vi "ROOT - Restore Session Defaults.vi"(0 "Session Handle in":T1, 11 "error in (no error)":errorcluster) -> (4 "Session Handle out":T1, 15 "error out":errorcluster)   [LabVIEW 2017, in "Session - Root.lvclass"]
doc: "Initializes a measurement session\n\nSession data is set to the default values from \"set Defaults.vi\""
uses:
  Session - Root.lvclass
  Typedefs/Session Handle.ctl
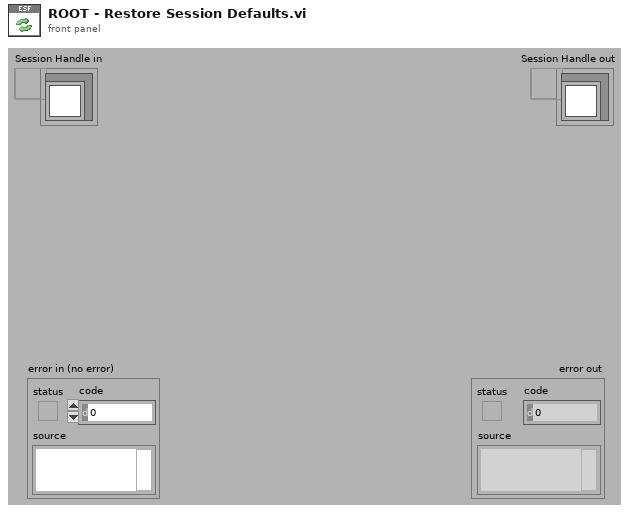
[diagram p1: front panel]
types:
  T1 = typedef "Session - Root.lvclass/Session Handle.ctl" = refnum<data-value>
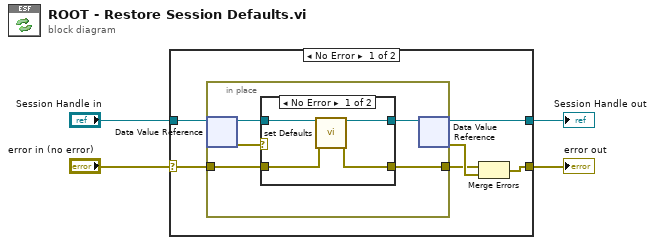
[diagram p0: block diagram]
diagram:
  n1 = case shown="No Error" "error in (no error)" {
    selector: "error in (no error)" -> [w8 w23]
    tunnel: "Session Handle in" -> [w10 w22]
    tunnel: [w9 w22] -> w3
    tunnel: [w5 w23] -> w1
    frame No Error {
      n2 = in-place {
        in-place-border: w8 -> [w12]
        in-place-border: [w11] -> w6
        n3 = in-place-dvr #1(w10) -> (w15:refnum<class "Session - Root.lvclass">, w13:errorcluster)
        n4 = case shown="No Error" w13 {
          tunnel: w15 -> [w19 w20]
          tunnel: [w18 w20] -> w14
          tunnel: w12 -> [w17 w21]
          tunnel: [w16 w21] -> w11
          frame No Error {
            n5 = call-dynamic "set Defaults.vi"("OBJ - Session in"=w19, "error in"=w17) -> ("OBJ - Session out"=w18:refnum<class "Session - Root.lvclass">, "error out"=w16:errorcluster)  [unwired: 12 in]
          }
          frame Error {
          }
        }
        n6 = in-place-dvr #1(w14) -> (w9:T1, w7:errorcluster)
      }
      n7 = Merge Errors(w6, w7) -> (w5:errorcluster)
    }
    frame Error {
    }
  }
  "error out" <- w1
  "Session Handle out" <- w3
